vi "Pre Launch Init.vi"(11 "Inspection Statemachine in":refnum<class "Inspection Statemachine.lvclass">) -> (0 "error out":errorcluster, 3 "Inspection Statemachine out":refnum<class "Inspection Statemachine.lvclass">)   [LabVIEW 2019, in "Inspection Statemachine.lvclass"]
doc: "(<B>Filename</B>: Actor Framework.lvlib:Actor.lvclass:Pre Launch Init.vi)\n\nDefines behavior that occurs after the Launch Nested Actor method is invoked but before the actor's Actor Core method begins running.\n\nBy default, this method does nothing. A descendant class may override it to define behavior."
uses:
  Inspection Statemachine.lvclass
  <vilib>/ActorFramework/Message Enqueuer/Message Enqueuer.lvclass
  <vilib>/vision/Image Controls.llb/IMAQ Image.ctl
  Common/Controls/Diagnostics Result.ctl
  Common/Controls/Acknowledgement.ctl
  Common/Controls/Camera Optics Diagnostics Result.ctl
  Controls/Result Cluster_SM.ctl
  Common/Controls/Pop-up Input.ctl
  Common/Controls/AllPartInfo.ctl
  <vilib>/ActorFramework/Actor/Actor.lvclass
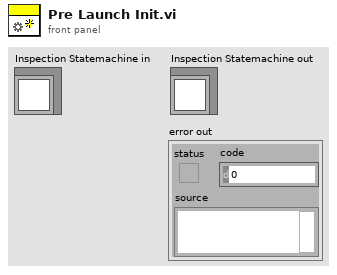
[diagram p1: front panel]
types:
  T1 = typedef "IMAQ Image.ctl" = refnum<image>
  T2 = typedef "AllPartInfo.ctl" = cluster{"PartName":string, "NumberOfRacks":u8, "MeasurementIDsArray":u16[], "MeasurementNamesArray":string[], "SpecValuesArray":cluster{"LCL":dbl, "UCL":dbl, "LSL":dbl, "USL":dbl, "NominalValue":dbl}[]}[]
  T3 = cluster{"PartName":string, "RackID":u8, "Initialize":bool, "MeasurementIDsArray":u16[], "MeasurementNamesArray":string[], "SpecValuesArray":cluster{"LCL":dbl, "UCL":dbl, "LSL":dbl, "USL":dbl, "NominalValue":dbl}[], "CameraNamesArray":string[]}
  T4 = typedef "Inspection Statemachine.lvclass/Result Cluster_SM.ctl" = cluster{"RackID":u8, "MeasurementValuesArray ":dbl[], "ImagesArray":T1[], "ResultPF":bool, "ProductionCountDetails":cluster{"TotalFail":u64, "TotalPass":u64, "TotalCount":u64}, "ReelCountDetails":cluster{"ReelFail":u64, "ReelPass":u64, "ReelCount":u64}, "ControlPFArray":bool[], "SpecificationPFArray":bool[], "SpecificationFail":bool, "ReelNumber":u64, "Status":string}
  T5 = typedef "Pop-up Input.ctl" = cluster{"Pop-up Type":enum16{"Open Logo Display", "Close Logo Display", "Open Loading Bar", "Close Loading Bar", "Open Alert Display", "Close Alert Display", "One button dialog box", "Two button dialog box", "User Authentication"}, "Title":string, "Message":string, "Button 1 Text":string, "Button 2 Text":string, "Show Close? T/F":bool, "Title Blink? T/F":bool, "Title Blink Colour":u32}
  T6 = typedef "Camera Optics Diagnostics Result.ctl" = cluster{"LightCameraName":string, "DiagnosedImage":T1, "DustPercentage":dbl, "Result":bool}
  T7 = typedef "Diagnostics Result.ctl" = cluster{"Result":bool, "StateMessage":string}
  T8 = cluster{"PartName":string, "ConnectorsInReel":u64, "TotalCount":u64, "OperatorName":string, "StampingMachineID":u8}
  T9 = typedef "Acknowledgement.ctl" = cluster{"Enqueuer":refnum<class "Message Enqueuer.lvclass">, "VIReference":refnum<vi>, "VIName":string}
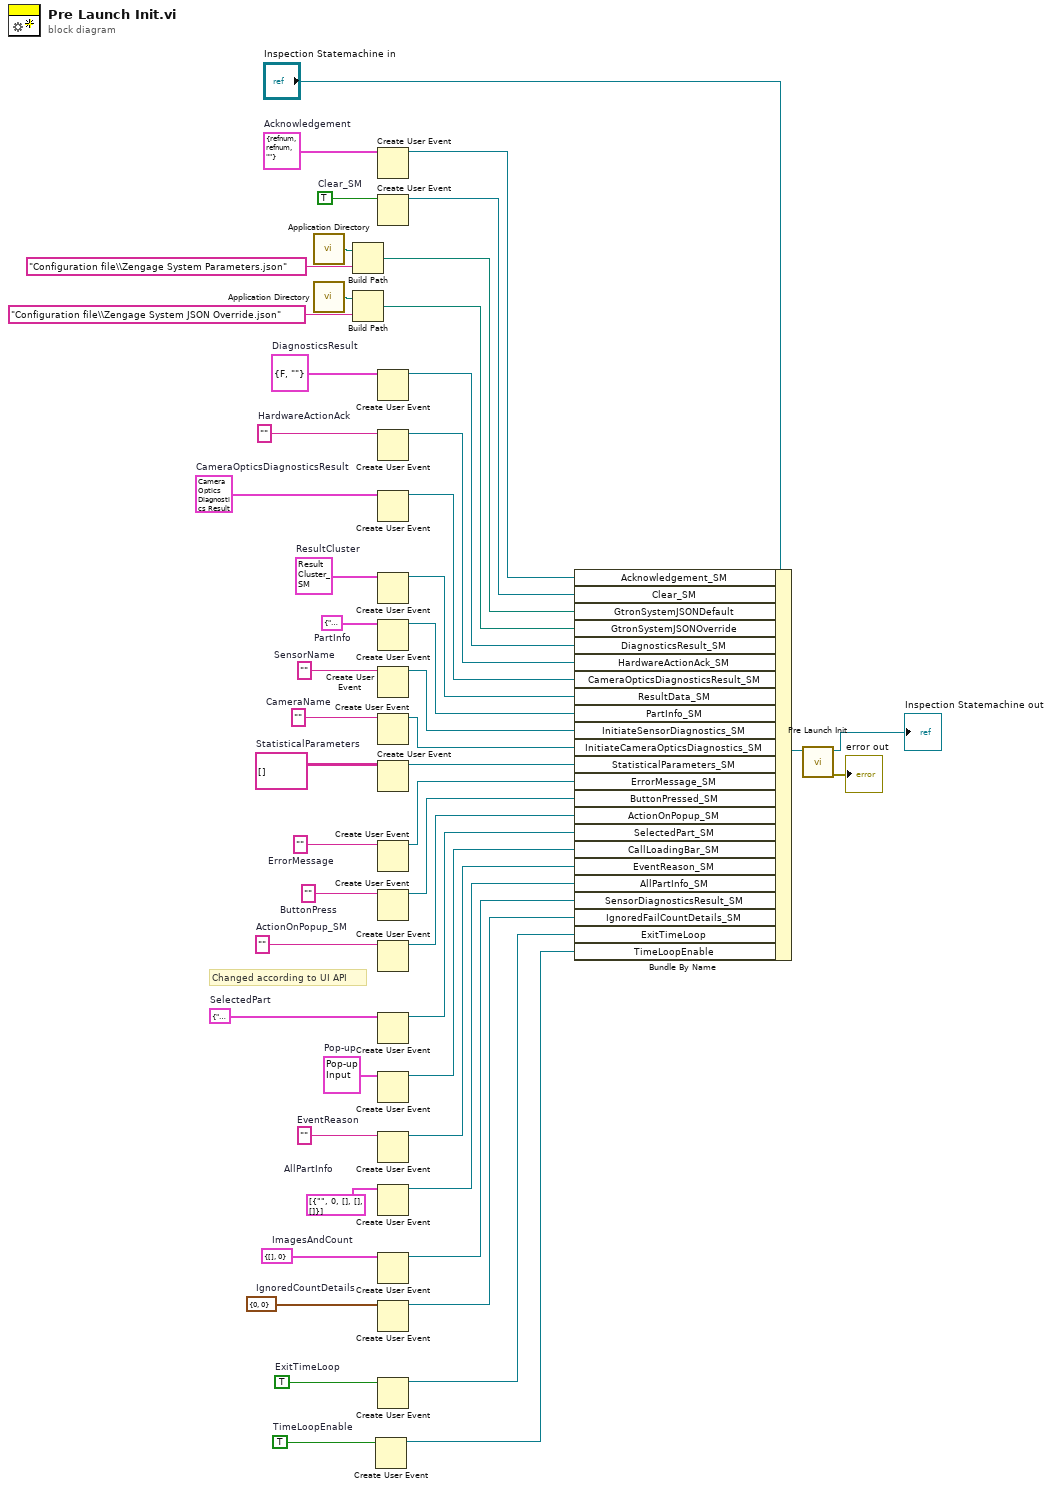
[diagram p0: block diagram]
diagram:
  w2 = TRUE  # TimeLoopEnable
  w4 = TRUE  # ExitTimeLoop
  w6 = cluster{"ReelCount":u64, "TotalCount":u64} {"ReelCount"=0, "TotalCount"=0}  # IgnoredCountDetails
  w8 = cluster{"Image Array":T1[], "ImageCount":u64} {"Image Array"=[], "ImageCount"=0}  # ImagesAndCount
  w26 = string[][] []  # StatisticalParameters
  w10 = T2 [{"PartName"="", "NumberOfRacks"=0, "MeasurementIDsArray"=[], "MeasurementNamesArray"=[], "SpecValuesArray"=[]}]  # AllPartInfo
  w28 = T3 {"PartName"="", "RackID"=0, "Initialize"=FALSE, "MeasurementIDsArray"=[], "MeasurementNamesArray"=[], "SpecValuesArray"=[], "CameraNamesArray"=[]}  # PartInfo
  w30 = T4 {"RackID"=0, "MeasurementValuesArray "=[], "ImagesArray"=[], "ResultPF"=FALSE, "ProductionCountDetails"={"TotalFail"=0, "TotalPass"=0, "TotalCount"=0}, "ReelCountDetails"={"ReelFail"=0, "ReelPass"=0, "ReelCount"=0}, "ControlPFArray"=[], "SpecificationPFArray"=[], "SpecificationFail"=FALSE, "ReelNumber"=0, "Status"=""}  # ResultCluster
  w42 = ""  # HardwareActionAck
  w22 = ""  # EventReason
  w23 = ""  # ActionOnPopup_SM
  w24 = T5 {"Pop-up Type"=enum."Open Logo Display", "Title"="", "Message"="", "Button 1 Text"="", "Button 2 Text"="", "Show Close? T/F"=FALSE, "Title Blink? T/F"=FALSE, "Title Blink Colour"=0}  # Pop-up
  w27 = ""  # CameraName
  w31 = T6 {"LightCameraName"="", "DiagnosedImage"=refnum, "DustPercentage"=0.0, "Result"=TRUE}  # CameraOpticsDiagnosticsResult
  w33 = T7 {"Result"=FALSE, "StateMessage"=""}  # DiagnosticsResult
  w40 = ""  # SensorName
  w41 = ""  # ErrorMessage
  w43 = T8 {"PartName"="", "ConnectorsInReel"=0, "TotalCount"=0, "OperatorName"="", "StampingMachineID"=0}  # SelectedPart
  w46 = TRUE  # Clear_SM
  w47 = T9 {"Enqueuer"=refnum, "VIReference"=refnum, "VIName"=""}  # Acknowledgement
  w48 = ""  # ButtonPress
  # "Changed according to UI API"
  n1 = call <vilib>:"Application Directory.vi"() -> ("Application Directory"=w45:path)
  n2 = call <vilib>:"Application Directory.vi"() -> ("Application Directory"=w35:path)
  n3 = Build Path(base path=w45, name or relative path="Configuration file\\Zengage System Parameters.json") -> (appended path=w37:path)
  n4 = Build Path(base path=w35, name or relative path="Configuration file\\Zengage System JSON Override.json") -> (appended path=w34:path)
  n5 = Create User Event(user event datatype=w2) -> (user event=w1:refnum<user-event>)  [unwired: 1 in, 1 out]
  n6 = Create User Event(user event datatype=w47) -> (user event=w39:refnum<user-event>)  [unwired: 1 in, 1 out]
  n7 = Create User Event(user event datatype=w46) -> (user event=w38:refnum<user-event>)  [unwired: 1 in, 1 out]
  n8 = Create User Event(user event datatype=w33) -> (user event=w11:refnum<user-event>)  [unwired: 1 in, 1 out]
  n9 = Create User Event(user event datatype=w42) -> (user event=w32:refnum<user-event>)  [unwired: 1 in, 1 out]
  n10 = Create User Event(user event datatype=w31) -> (user event=w13:refnum<user-event>)  [unwired: 1 in, 1 out]
  n11 = Create User Event(user event datatype=w30) -> (user event=w29:refnum<user-event>)  [unwired: 1 in, 1 out]
  n12 = Create User Event(user event datatype=w28) -> (user event=w19:refnum<user-event>)  [unwired: 1 in, 1 out]
  n13 = Create User Event(user event datatype=w40) -> (user event=w18:refnum<user-event>)  [unwired: 1 in, 1 out]
  n14 = Create User Event(user event datatype=w27) -> (user event=w17:refnum<user-event>)  [unwired: 1 in, 1 out]
  n15 = Create User Event(user event datatype=w26) -> (user event=w16:refnum<user-event>)  [unwired: 1 in, 1 out]
  n16 = Create User Event(user event datatype=w41) -> (user event=w15:refnum<user-event>)  [unwired: 1 in, 1 out]
  n17 = Create User Event(user event datatype=w48) -> (user event=w25:refnum<user-event>)  [unwired: 1 in, 1 out]
  n18 = Create User Event(user event datatype=w23) -> (user event=w14:refnum<user-event>)  [unwired: 1 in, 1 out]
  n19 = Create User Event(user event datatype=w43) -> (user event=w20:refnum<user-event>)  [unwired: 1 in, 1 out]
  n20 = Create User Event(user event datatype=w24) -> (user event=w12:refnum<user-event>)  [unwired: 1 in, 1 out]
  n21 = Create User Event(user event datatype=w22) -> (user event=w21:refnum<user-event>)  [unwired: 1 in, 1 out]
  n22 = Create User Event(user event datatype=w10) -> (user event=w9:refnum<user-event>)  [unwired: 1 in, 1 out]
  n23 = Create User Event(user event datatype=w8) -> (user event=w7:refnum<user-event>)  [unwired: 1 in, 1 out]
  n24 = Create User Event(user event datatype=w6) -> (user event=w5:refnum<user-event>)  [unwired: 1 in, 1 out]
  n25 = Create User Event(user event datatype=w4) -> (user event=w3:refnum<user-event>)  [unwired: 1 in, 1 out]
  n26 = Bundle By Name(cluster="Inspection Statemachine in", "Acknowledgement_SM"=w39, "Clear_SM"=w38, "GtronSystemJSONDefault"=w37, "GtronSystemJSONOverride"=w34, "DiagnosticsResult_SM"=w11, "HardwareActionAck_SM"=w32, "CameraOpticsDiagnosticsResult_SM"=w13, "ResultData_SM"=w29, "PartInfo_SM"=w19, "InitiateSensorDiagnostics_SM"=w18, "InitiateCameraOpticsDiagnostics_SM"=w17, "StatisticalParameters_SM"=w16, "ErrorMessage_SM"=w15, "ButtonPressed_SM"=w25, "ActionOnPopup_SM"=w14, "SelectedPart_SM"=w20, "CallLoadingBar_SM"=w12, "EventReason_SM"=w21, "AllPartInfo_SM"=w9, "SensorDiagnosticsResult_SM"=w7, "IgnoredFailCountDetails_SM"=w5, "ExitTimeLoop"=w3, "TimeLoopEnable"=w1) -> (w49:refnum<class "Inspection Statemachine.lvclass">)
  n27 = call-parent "Pre Launch Init.vi"("Actor in"=w49) -> ("error out"=→"error out":errorcluster, "Actor out"=→"Inspection Statemachine out":refnum<class "Inspection Statemachine.lvclass">)  [unwired: 9 in]
